vi "GetSingleMeasData.vi"(8 "error in (no error)":errorcluster, 11 "TCP Network Connection in":refnum<k5>) -> (0 "error out":errorcluster, 2 "Meas Result":dbl[](array[numeric]), 3 "TCP Network Connection out":refnum<k5>, 5 "Respond":string[](array[string]))   [LabVIEW 2017]
uses:
  AT901 API/TypeDefinitions/ES_DataType.ctl
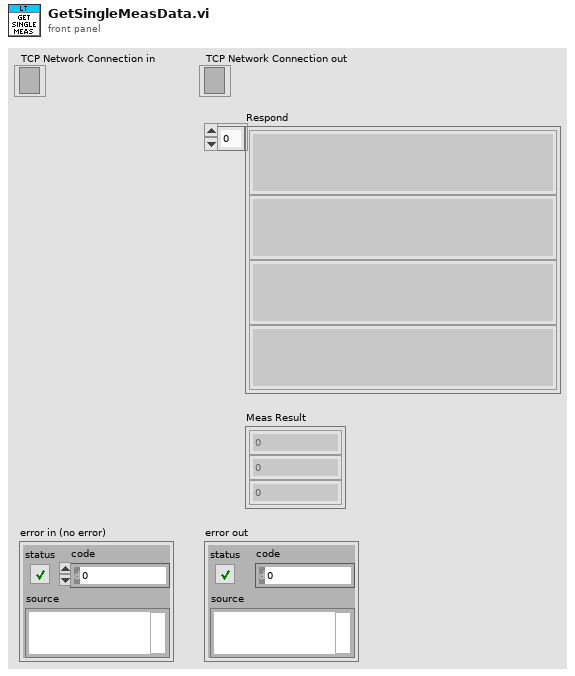
[diagram p1: front panel]
types:
  T1 = typedef "ES_DataType.ctl" = enum32{"ES_DT_Command", "ES_DT_Error", "ES_DT_SingleMeasResult", "ES_DT_MultiMeasResult", "ES_DT_StationaryProbeMeasResult", "ES_DT_ContinuousProbeMeasResult", "ES_DT_NivelResult", "ES_DT_ReflectorPosResult", "ES_DT_SystemStatusChange", "ES_DT_SingleMeasResult2", "ES_DT_MultiMeasResult2", "ES_DT_ProbePosResult"}
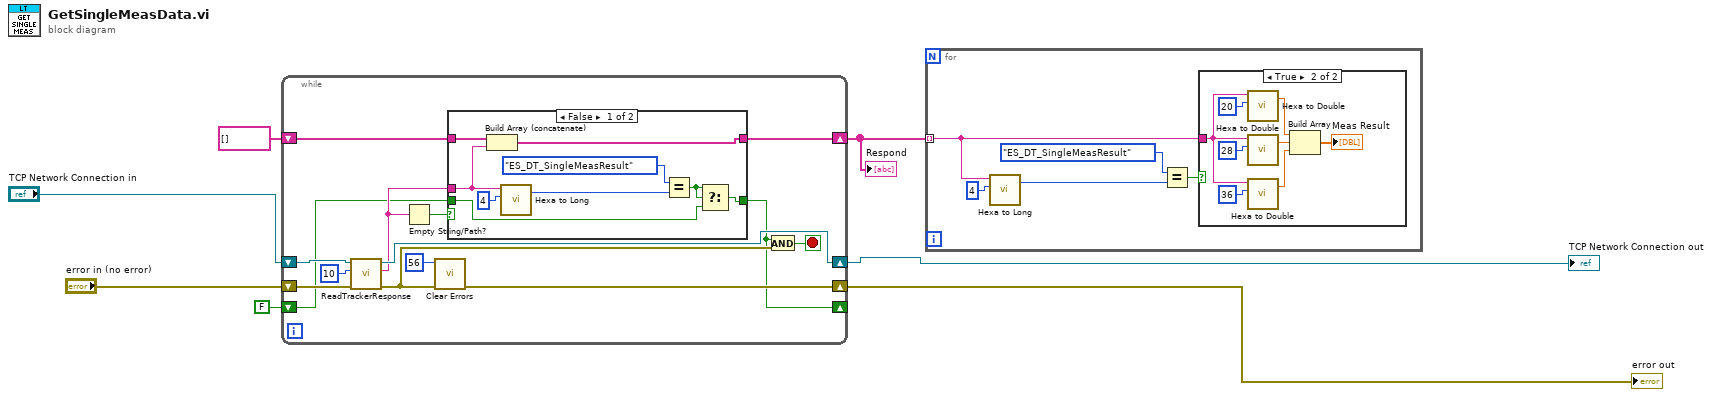
[diagram p0: block diagram]
diagram:
  n1 = while {
    shift-right: [w20] -> w4
    shift-left: "TCP Network Connection in" -> [w21]
    shift-right: [w15] -> w3
    shift-left: "error in (no error)" -> [w19]
    shift-right: [w11] -> w5
    shift-left: string[] [] -> [w10]
    shift-right: [w8] -> _
    shift-left: FALSE ("logical AND") -> [w9]
    stop <- w17 stop-if-true
    n2 = call "ReadTrackerResponse.vi"("error in"=w19, "timeout ms (1000)"=10, "connection ID in"=w21) -> ("error out"=w16:errorcluster, "Tracker Response"=w12:string, "connection ID out"=w20:refnum<k5>)  [unwired: 6 in]
    n3 = Empty String/Path?(string/path=w12) -> (empty?=w13:bool)
    n4 = call <vilib>:"Clear Errors.vi"("error in (no error)"=w16, "specific error code to clear (0: all)"=56) -> ("error out"=w15:errorcluster)  [unwired: 4 in, 1 out]
    n5 = case shown="False" w13 {
      tunnel: w12 -> [w23 _]
      tunnel: [w30 w32] -> w11
      tunnel: w10 -> [w29 w32]
      tunnel: w9 -> [w28 w31]
      tunnel: [w27 w31] -> w8
      frame False {
        n6 = Build Array (concatenate)(w29, w23) -> (w30:string[])
        n7 = call "Hexa to Long.vi"("Hexa"=w23, "Index"=4) -> ("Long"=w25:u32)  [unwired: 4 in]
        n8 = Equal?(x=ES_DataType."ES_DT_SingleMeasResult" ("ES_DataType"), y=w25) -> (x = y?=w22:bool)
        n9 = Select(t=w22, s=w22, f=w28) -> (s? t:f=w27:bool)
      }
      frame True {
      }
    }
    n10 = And(x=w8, y=w16) -> (x .and. y?=w17:bool)
  }
  "Respond" <- w5
  "TCP Network Connection out" <- w4
  "error out" <- w3
  n11 = for {
    tunnel: w5 -> [w37] mode=indexing
    n12 = call "Hexa to Long.vi"("Hexa"=w37, "Index"=4) -> ("Long"=w35:u32)  [unwired: 4 in]
    n13 = Equal?(x=ES_DataType."ES_DT_SingleMeasResult" ("ES_DataType"), y=w35) -> (x = y?=w34:bool)
    n14 = case shown="True" w34 {
      tunnel: w37 -> [_ w42]
      frame False {
      }
      frame True {
        n15 = call "Hexa to Double.vi"("Hexa"=w42, "Index"=20) -> ("Double"=w39:dbl)  [unwired: 4 in]
        n16 = call "Hexa to Double.vi"("Hexa"=w42, "Index"=28) -> ("Double"=w40:dbl)  [unwired: 4 in]
        n17 = call "Hexa to Double.vi"("Hexa"=w42, "Index"=36) -> ("Double"=w41:dbl)  [unwired: 4 in]
        n18 = Build Array(w39, w40, w41) -> (→"Meas Result":dbl[])
      }
    }
  }
